vi "RSZVB Load Balanced Port Circuit Model Data.vi"(5 "Logical Port Number (1)":i32=1, 6 "Parameter (0: Port 1)":i32(ring) items=["Port 1", "Port 2"], 7 "File Name":string, 8 "error in (no error)":errorcluster {"code" format="%.0x"}, 9 "Function Type (0: Deembedding)":i32(ring) items=["Deembedding", "Embedding"], 10 "Channel (1)":i32=1, 11 "VISA session":refnum<visa-resource-name>) -> (0 "error out":errorcluster {"code" format="%.0x"}, 3 "dup VISA session":refnum<visa-resource-name>)   [LabVIEW 2011]
doc: "This VI loads data from a specified Touchstone file defining the characteristics of the current embedded/deembedded balanced port circuit model. A balanced port circuit model involving file import must be selected before using this VI. \n\nRemote-control command(s):\nMMEMory:LOAD:VNETworks<Ch>:BALanced:EMBedding<Log_pt> '<file_name>', PMAin | PSECondary \n\nMMEMory:LOAD:VNETworks<Ch>:BALanced:DEEMbedding<Log_pt> '<file_name>', PMAin | PSECondary"
uses:
  _utility/RSZVB Global Data.vi
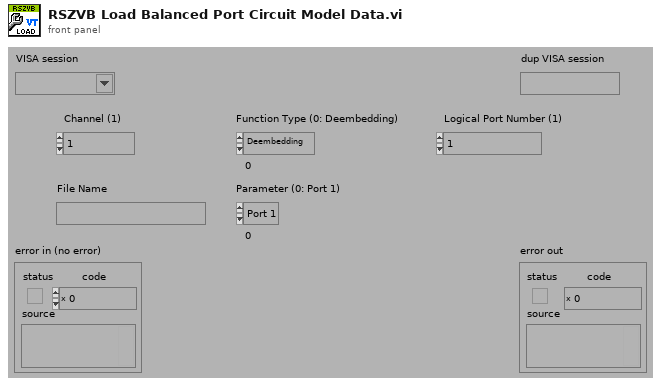
[diagram p1: front panel]
types:
  T1 = cluster{"Error Checking (T: On)":bool, "Installed Options":string[], "Data Valid?":bool, "Ports":i32, "Model":string[], "Option Checking (T: On)":bool}[]
  T2 = cluster{"Error Checking (T: On)":bool, "Installed Options":string[], "Data Valid?":bool, "Ports":i32, "Model":string[], "Option Checking (T: On)":bool}
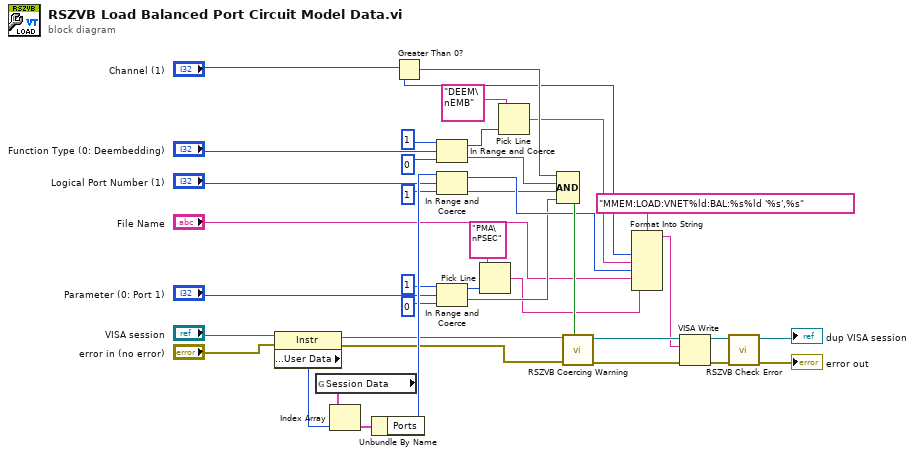
[diagram p0: block diagram]
diagram:
  n1 = property class="Instr"(reference="VISA session", error in="error in (no error)") -> (reference out=w27:refnum<visa-resource-name>, error out=w28:errorcluster, "General Settings:User Data"=w32:u32)
  n2 = global read "RSZVB Global Data.vi" "Session Data"() -> (w31:T1)
  n3 = Index Array(array=w31, index=w32) -> (element=w30:T2)
  n4 = Unbundle By Name(w30) -> ("Ports"=w29:i32)
  n5 = Greater Than 0?(x="Channel (1)") -> (x > 0?=w24:bool)
  n6 = In Range and Coerce(upper limit=1 ("lower limit"), x="Function Type (0: Deembedding)", lower limit=0) -> (coerced(x)=w18:i32, In Range?=w21:bool)
  n7 = In Range and Coerce(upper limit=w29, x="Logical Port Number (1)", lower limit=1) -> (coerced(x)=w20:i32, In Range?=w16:bool)
  n8 = In Range and Coerce(upper limit=1 ("lower limit"), x="Parameter (0: Port 1)", lower limit=0) -> (coerced(x)=w12:i32, In Range?=w11:bool)
  n9 = Pick Line(multi-line string="PMA\nPSEC", line index=w12) -> (output string=w1:string)  [unwired: 1 in]
  n10 = Pick Line(multi-line string="DEEM\nEMB", line index=w18) -> (output string=w17:string)  [unwired: 1 in]
  n11 = Compound Arithmetic op=AND(w24, w21, w16, w11) -> (w23:bool)
  n12 = call "RSZVB Coercing Warning.vi"("In Range?"=w23, "error in (no error)"=w28, "VISA session"=w27) -> ("error out"=w37:errorcluster, "dup VISA session"=w38:refnum<visa-resource-name>)  [unwired: 7 in]
  n13 = Format Into String(format string="MMEM:LOAD:VNET%ld:BAL:%s%ld '%s',%s", "Channel (1)", w17, w20, "File Name", w1) -> (resulting string=w33:string)  [unwired: 2 in, 1 out]
  n14 = VISA Write(VISA resource name=w38, write buffer=w33, error in (no error)=w37) -> (VISA resource name out=w35:refnum<visa-resource-name>, error out=w36:errorcluster)  [unwired: 1 out]
  n15 = call "RSZVB Check Error.vi"("error in (no error)"=w36, "VISA session"=w35) -> ("error out"=→"error out":errorcluster, "dup VISA session"=→"dup VISA session":refnum<visa-resource-name>)  [unwired: 8 in]
